vi "GetChain.vi"(8 "error in (no error)":errorcluster) -> (0 "error out":errorcluster, 3 "Chain OF Handler":refnum<class "ErrorHandler(Handler).lvclass">)   [LabVIEW 2014, in "Chain Of Responsibility Pattern.lvlib"]
uses:
  Chain Of Responsibility Pattern.lvlib
  ErrorHandler(Handler)_class/ErrorHandler(Handler).lvclass
  Handler/Level1Handler_class/Level1Handler.lvclass
  Handler/Level2Handler_class/Level2Handler.lvclass
  Handler/Level3Handler_class/Level3Handler.lvclass
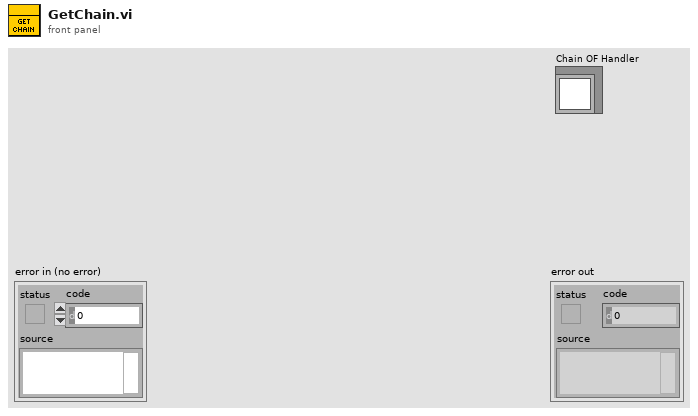
[diagram p1: front panel]
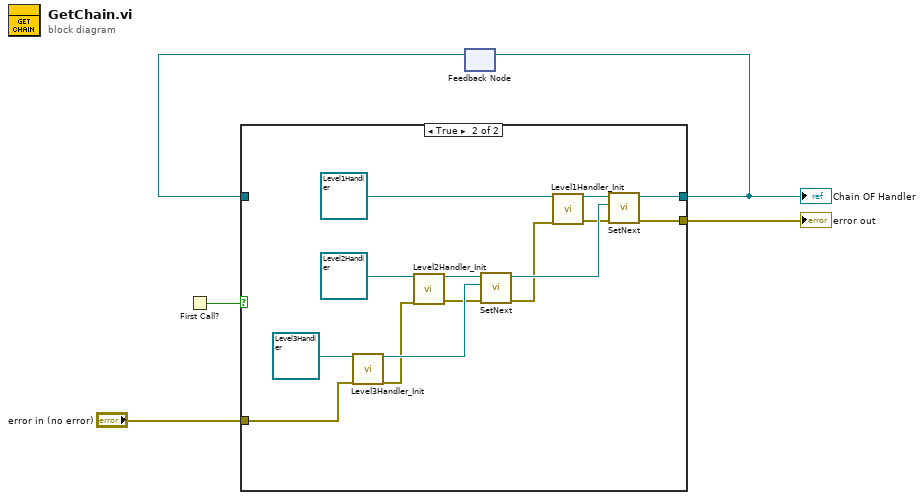
[diagram p0: block diagram]
diagram:
  n1 = First Call?() -> (First Call?: T/F=w3:bool)
  n2 = feedback #1() -> (w1:refnum<class "Level1Handler.lvclass">)  [unwired: 1 in]
  n3 = case shown="True" w3 {
    tunnel: "error in (no error)" -> [w6 w10]
    tunnel: [w6 w9] -> w4
    tunnel: [w7 w8] -> w2
    tunnel: w1 -> [w7 _]
    frame False {
    }
    frame True {
      n4 = call "Level3Handler_Init.vi"("object in"=refnum<class "Level3Handler.lvclass"> refnum ("Level3Handler"), "error in (no error)"=w10) -> ("object out"=w16:refnum<class "Level3Handler.lvclass">, "error out"=w14:errorcluster)  [unwired: 16 in]
      n5 = call "Level2Handler_Init.vi"("object in"=refnum<class "Level2Handler.lvclass"> refnum ("Level2Handler"), "error in (no error)"=w14) -> ("object out"=w17:refnum<class "Level2Handler.lvclass">, "error out"=w13:errorcluster)  [unwired: 16 in]
      n6 = call "SetNext.vi"("error in (no error)"=w13, "Next"=w16, "ErrorHandler(Handler) in"=w17) -> ("error out"=w12:errorcluster, "ErrorHandler(Handler) out"=w15:refnum<class "Level2Handler.lvclass">)  [unwired: 7 in]
      n7 = call "Level1Handler_Init.vi"("object in"=refnum<class "Level1Handler.lvclass"> refnum ("Level1Handler"), "error in (no error)"=w12) -> ("object out"=w18:refnum<class "Level1Handler.lvclass">, "error out"=w11:errorcluster)  [unwired: 16 in]
      n8 = call "SetNext.vi"("error in (no error)"=w11, "Next"=w15, "ErrorHandler(Handler) in"=w18) -> ("error out"=w9:errorcluster, "ErrorHandler(Handler) out"=w8:refnum<class "Level1Handler.lvclass">)  [unwired: 7 in]
    }
  }
  "error out" <- w4
  "Chain OF Handler" <- w2
  n9 = feedback-in #1(w2) -> ()
